vi "Chain4.vi"(7 "Name (\"\" to Use UUID)":string="CSM-Module") -> ()   [LabVIEW 2017, in "CSM-Testcase.lvlib"]
doc: "Creates a template for a CSM module without a user interface.\n\n> [!NOTE] CSM Name Rules\n> - The CSM module name must be unique to avoid entering the \"Critical Error\" state.\n> - If the input is \"\", a UUID will be used as the module name. This module will operate in independent mode and will not be listed in the module list.\n> - If the input ends with '#', the module will run in work mode. Modules with the same name will share the same message queue. External messages will be handled by the idle module.\n\n> [!NOTE] CSM Initialization State\n> - The default value is \"Macro: Initialize\", consistent with the JKISM state machine.\n> - This state is typically not modified and is provided to facilitate external programmatic changes to the initialization state.\n\n\n-- <b>Controls</b> --\n- <b>Name (\"\" to Use UUID)</b>: CSM Module Name\n- <b>Init State(\"Macro: Initialize\")</b>: Initialization State, default is \"Macro: Initialize\""
uses:
  CSM-Testcase.lvlib
  src/user.lib/_NEVSTOP/Communicable State Machine(CSM)/AdvanceAPI/CSM - Revert Arguments-Safe String.vi
  src/user.lib/_NEVSTOP/Communicable State Machine(CSM)/_Shared/Trim Single-line Text.vi
  src/user.lib/_NEVSTOP/Communicable State Machine(CSM)/AdvanceAPI/CSM - Make String Arguments Safe.vi
  src/user.lib/_NEVSTOP/Communicable State Machine(CSM)/AdvanceAPI/CSM - Break Down Multiple States String.vi
  src/user.lib/_NEVSTOP/Communicable State Machine(CSM)/AdvanceAPI/CSM - Keywords.vi
  src/user.lib/_NEVSTOP/Communicable State Machine(CSM)/_Polymophic/Build No-Reply Asynchronous Message with Arguments.vi
  src/user.lib/_NEVSTOP/Communicable State Machine(CSM)/_Polymophic/Build Asynchronous Message with Arguments.vi
  src/user.lib/_NEVSTOP/Communicable State Machine(CSM)/_Polymophic/Build Register Message.vi
  src/user.lib/_NEVSTOP/Communicable State Machine(CSM)/_Polymophic/Build Interrupt Broadcast Message.vi
  src/user.lib/_NEVSTOP/Communicable State Machine(CSM)/Communicable State Machine.lvlib
panel:
  out "Error Occurred":errorcluster
  out "State History":string
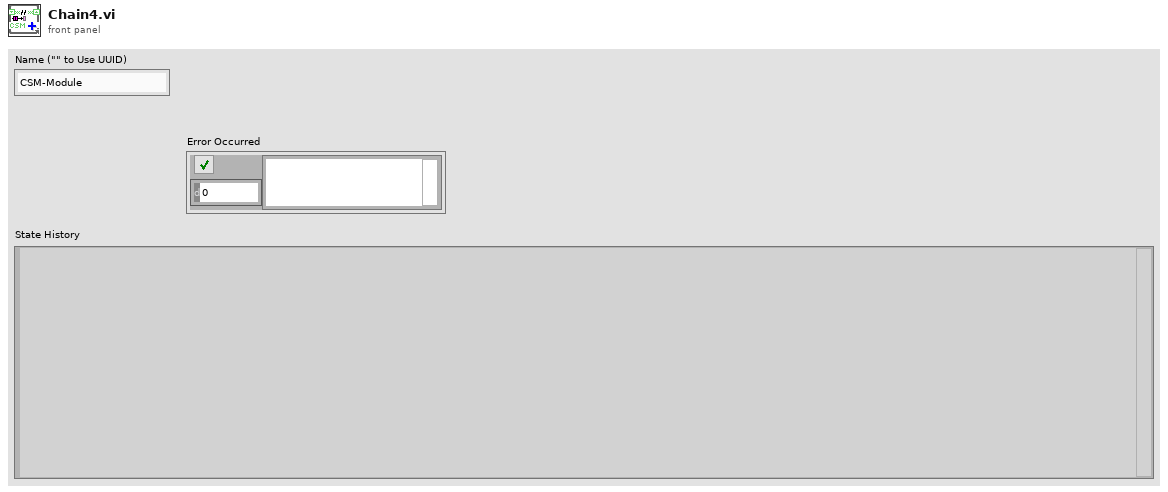
[diagram p1: front panel]
types:
  T1 = cluster{"Arguments":string, "Response":string, "error":errorcluster}
  T2 = enum32{"Invalid", "Standard", "Closed", "Hidden", "Minimized", "Maximized"}
  T3 = enum32{"invalid app kind", "Development System", "Run Time System", "Student Edition", "Embedded LabVIEW", "Evaluation", "Custom"}
  T4 = typedef "Communicable State Machine.lvlib/_CSM_Response Source Message.ctl" = cluster{"‘State":string, "’Arguments":string, "’Error":errorcluster}
  T5 = cluster{"Current VI Reference":refnum<vi>, "Close Panel on Exit?":bool}
  T6 = cluster{"Core":cluster{"Current VI Reference":refnum<vi>, "Close Panel on Exit?":bool}, "Your Boolean data":bool, "Your string data":string, "Counter":u32}
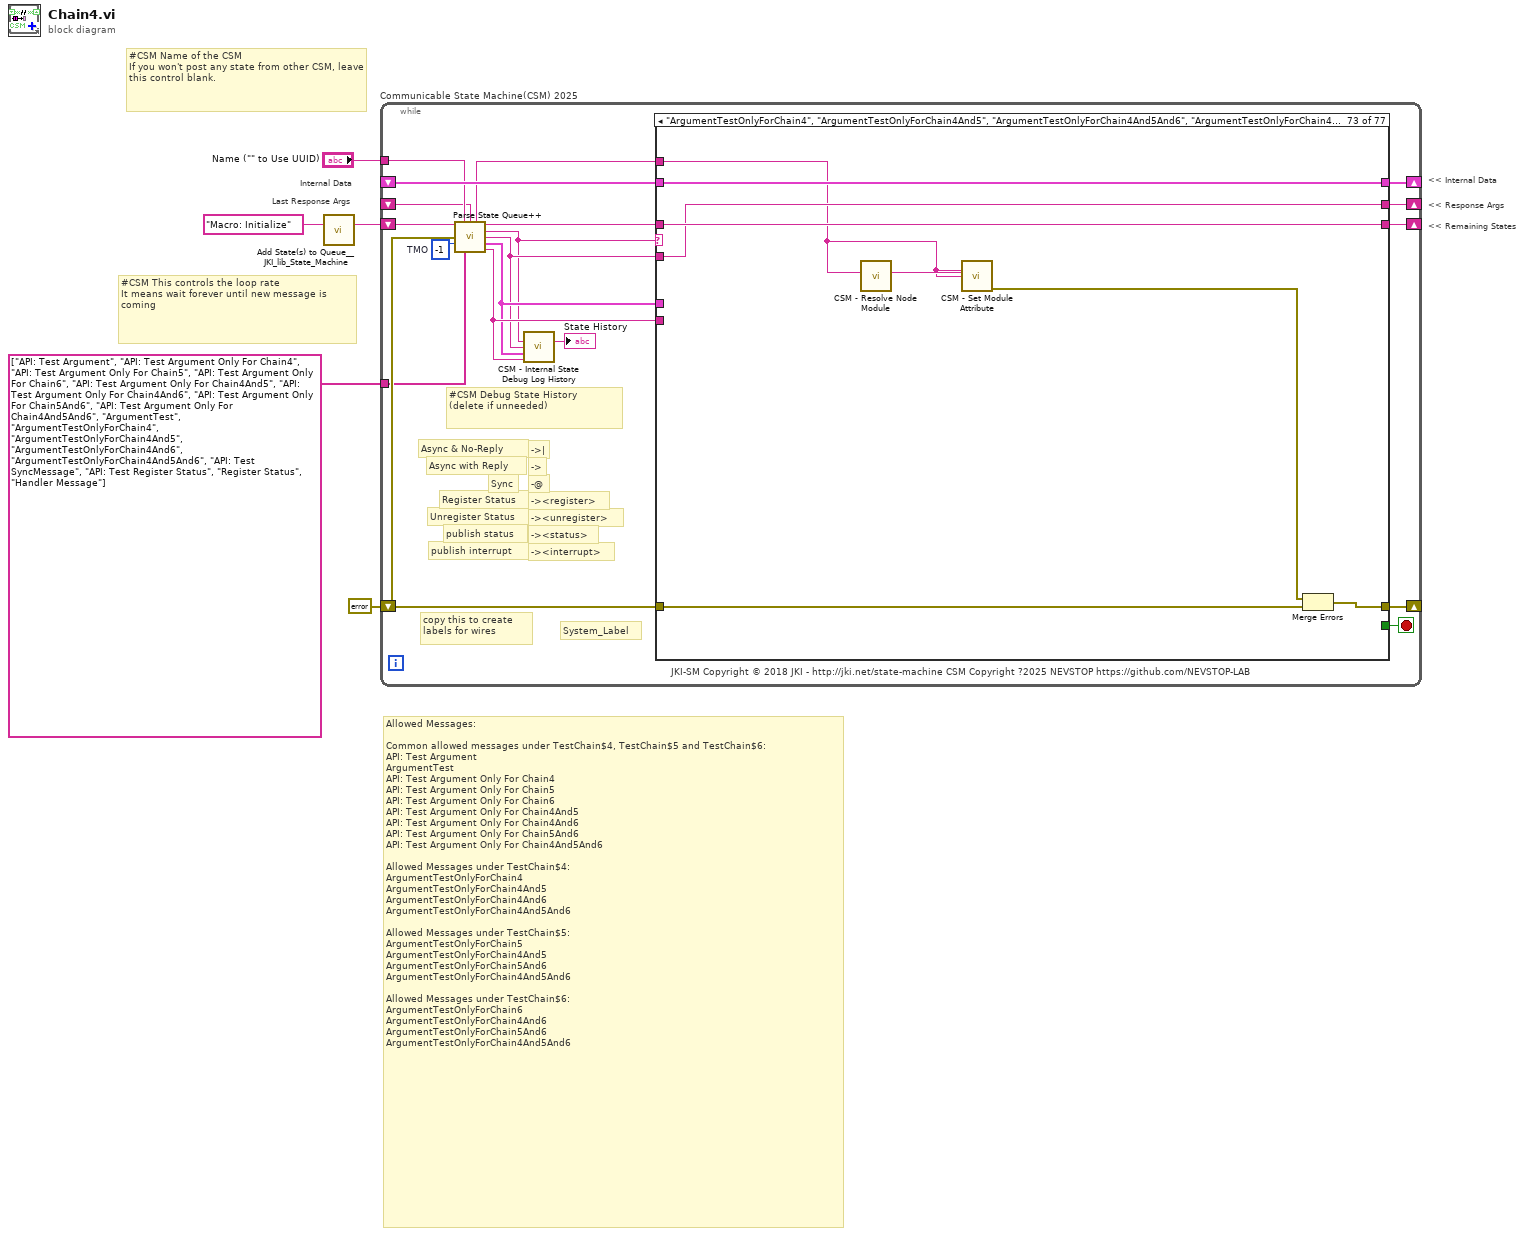
[diagram p0: block diagram]
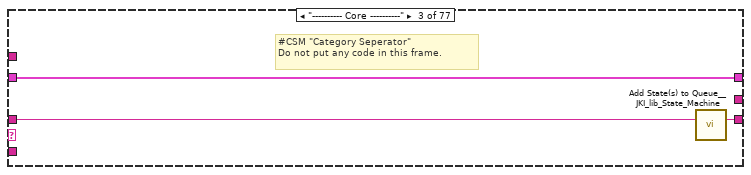
[diagram p4: hidden frame]
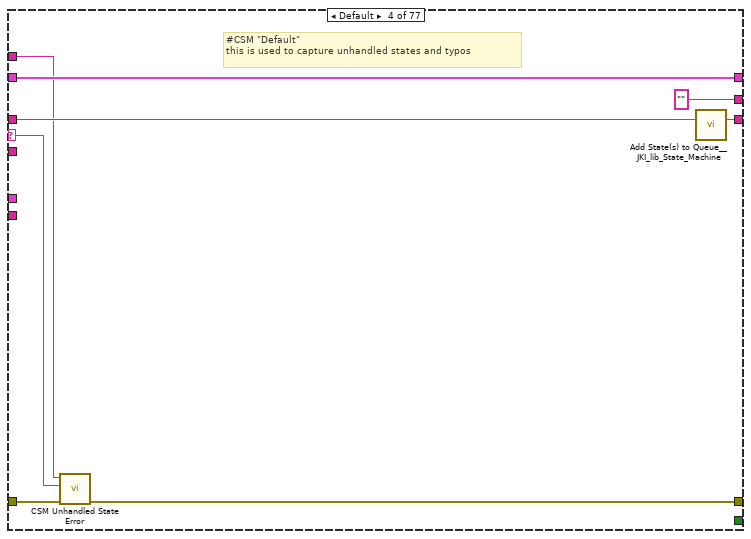
[diagram p5: hidden frame]
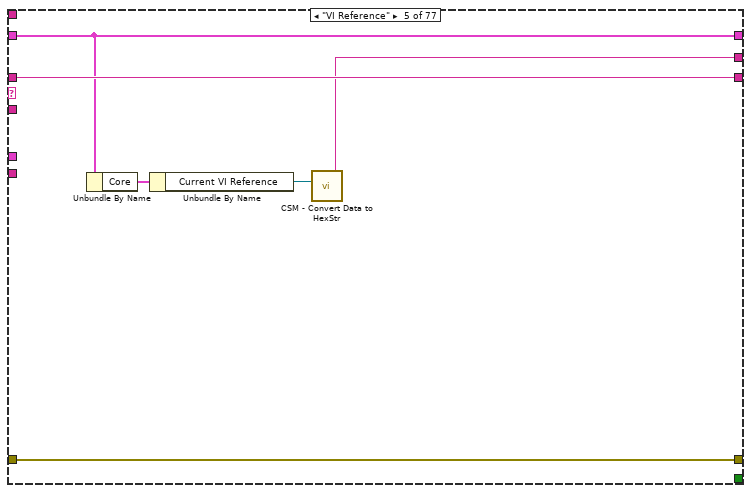
[diagram p6: hidden frame]
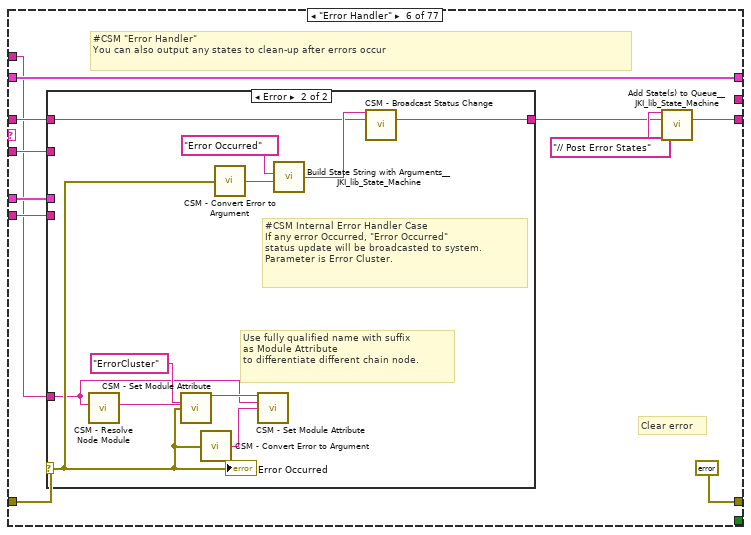
[diagram p7: hidden frame]
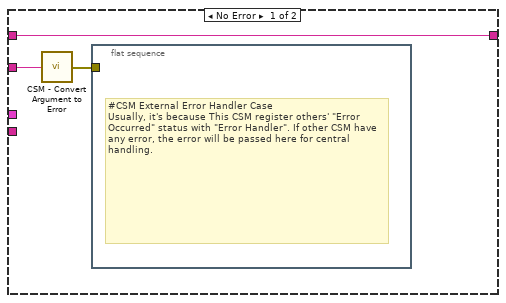
[diagram p8: hidden frame]
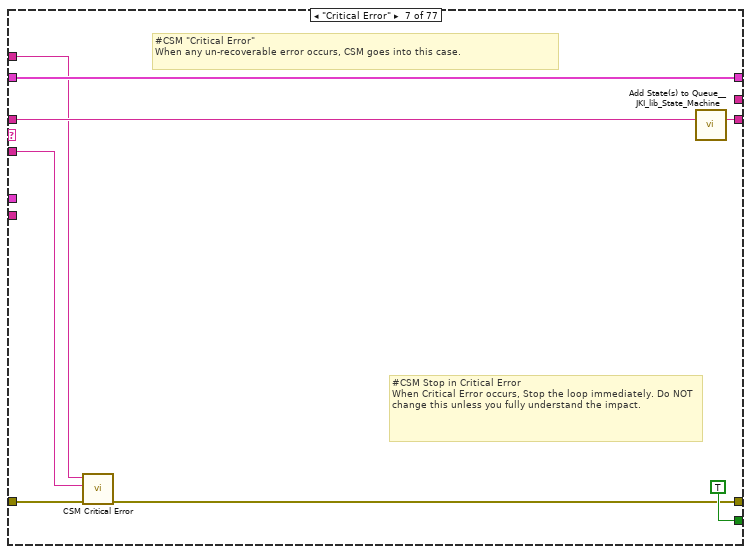
[diagram p9: hidden frame]
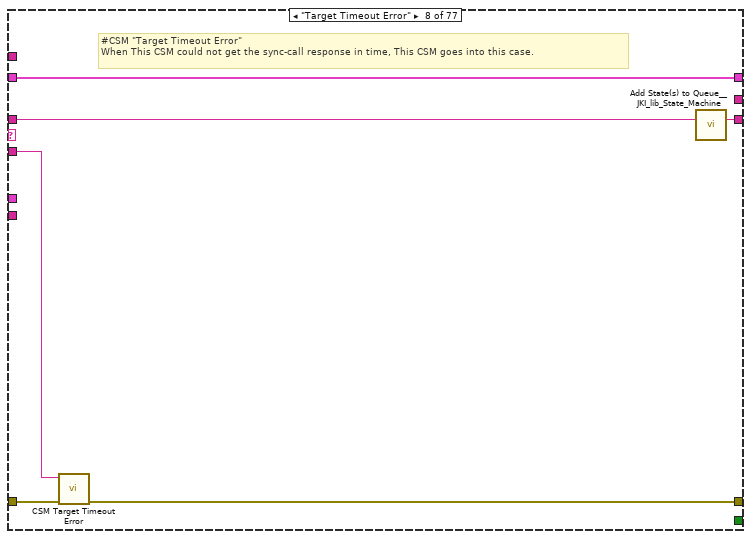
[diagram p10: hidden frame]
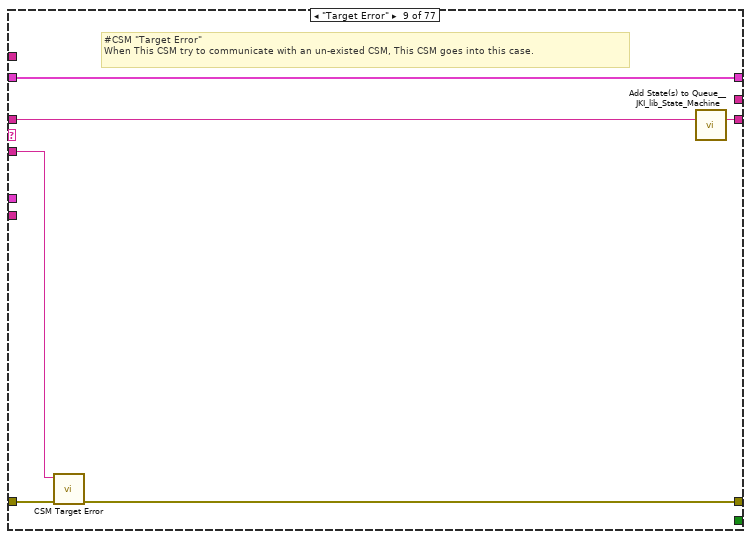
[diagram p11: hidden frame]
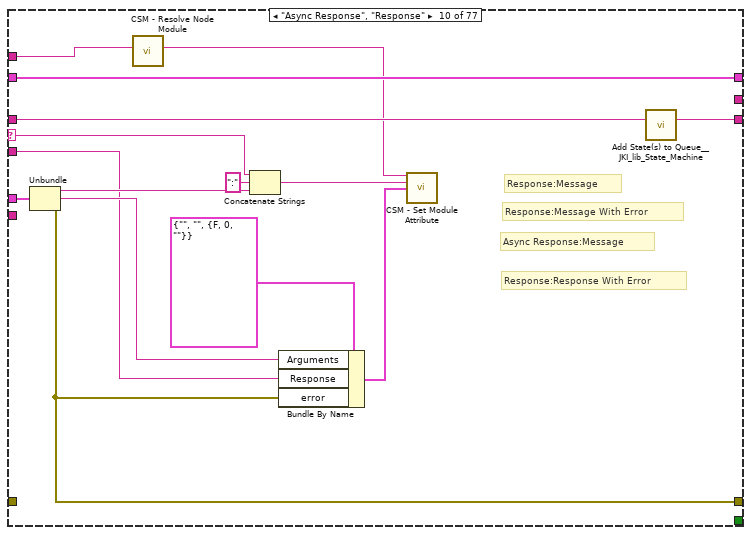
[diagram p12: hidden frame]
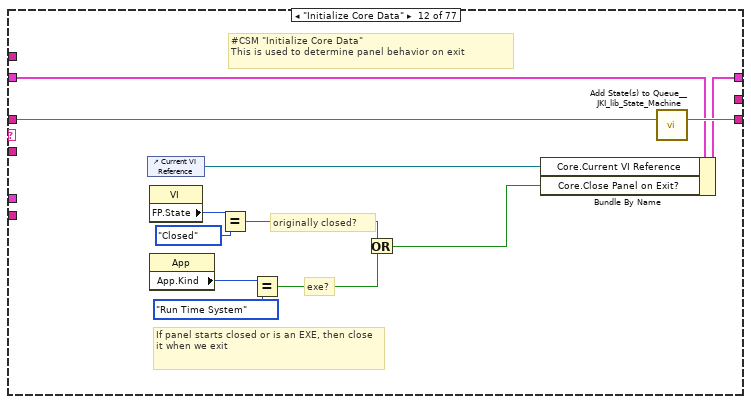
[diagram p14: hidden frame]
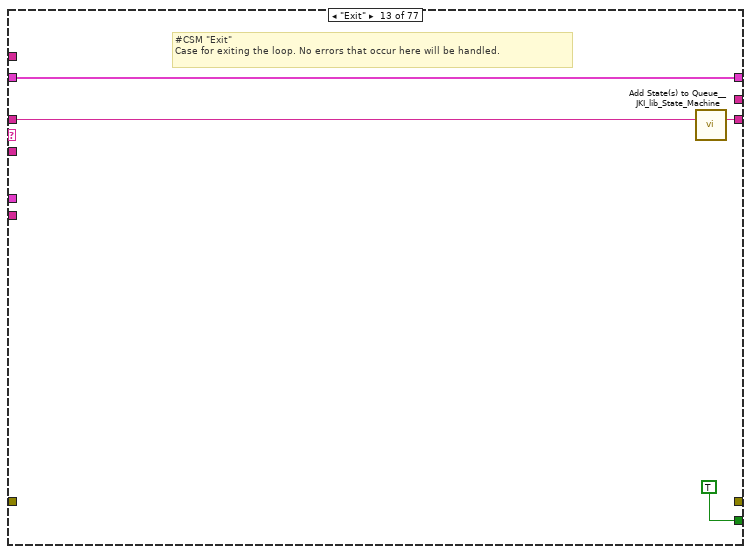
[diagram p15: hidden frame]
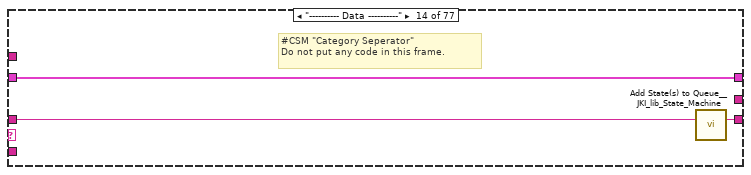
[diagram p16: hidden frame]
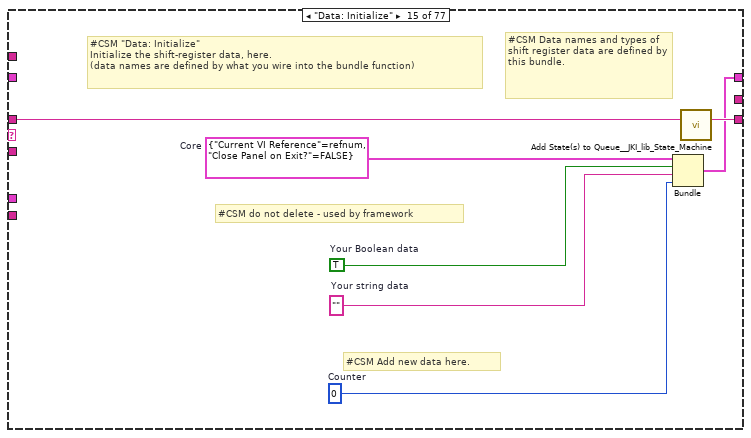
[diagram p17: hidden frame]
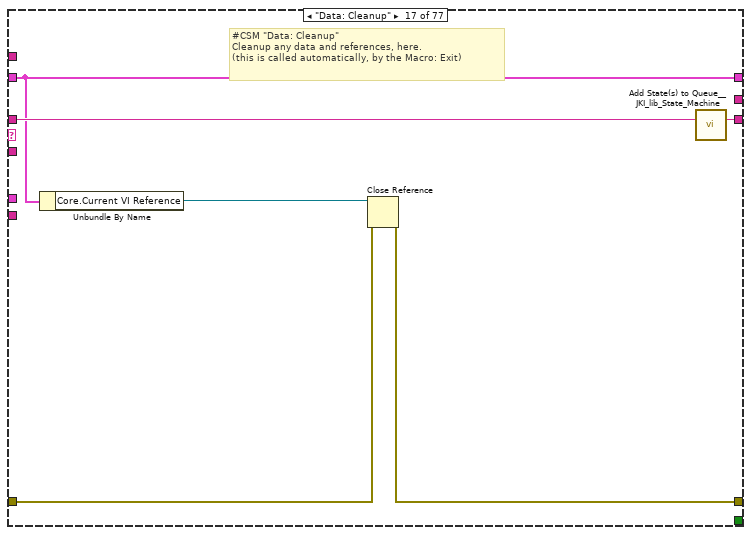
[diagram p19: hidden frame]
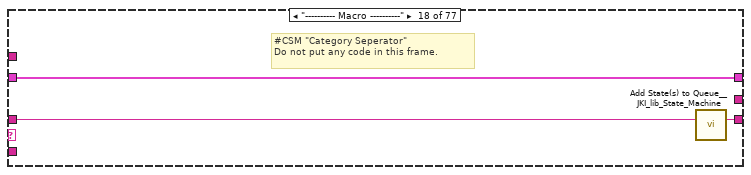
[diagram p20: hidden frame]
diagram:
  # "Allowed Messages:\n\nCommon allowed messages under TestChain$4, TestChain$5 and TestChain$6:\nAPI: Test Argument\nArgumentTest\nAPI: Test Argument Only For Chain4\nAPI: Test Argument Only For Chain5\nAPI: Test Argument Only For Chain6\nAPI: Test Argument Only For Chain4And5\nAPI: Test Argument Only For Chain4And6\nAPI: Test Argument Only For Chain5And6\nAPI: Test Argument Only For Chain4And5And6\n\nAllowed Messages under TestChain$4:\nArgumentTestOnlyForChain4\nArgumentTestOnlyForChain4And5\nArgumentTestOnlyForChain4And6\nArgumentTestOnlyForChain4And5And6\n\nAllowed Messages under TestChain$5:\nArgumentTestOnlyForChain5\nArgumentTestOnlyForChain4And5\nArgumentTestOnlyForChain5And6\nArgumentTestOnlyForChain4And5And6\n\nAllowed Messages under TestChain$6:\nArgumentTestOnlyForChain6\nArgumentTestOnlyForChain4And6\nArgumentTestOnlyForChain5And6\nArgumentTestOnlyForChain4And5And6"
  # "Last Response Args"
  # "Internal Data"
  # "#CSM Name of the CSM\nIf you won't post any state from other CSM, leave this control blank."
  # "#CSM This controls the loop rate\nIt means wait forever until new message is coming"
  # "<< Internal Data"
  # "<< Response Args"
  # "<< Remaining States"
  n1 = call <vilib>:"Add State(s) to Queue__JKI_lib_State_Machine.vi"("State(s) in (\"\")"="Macro: Initialize" ("Init State(\"Macro: Initialize\")")) -> ("States Out"=w5:string)  [unwired: 14 in]
  n2 = while "Communicable State Machine(CSM) 2025" {
    shift-right: [w19] -> _
    shift-left: _ -> [w18]
    shift-right: [w22] -> _
    shift-left: errorcluster {"status"=FALSE, "code"=0, "source"=""} ("error out") -> [w8]
    shift-right: [w21] -> _
    shift-left: w5 -> [w23]
    tunnel: "Name (\"\" to Use UUID)" -> [w15]
    shift-right: [w16] -> _
    shift-left: _ -> [w10]
    tunnel: string[] ["API: Test Argument", "API: Test Argument Only For Chain4", "API: Test Argument Only For Chain5", "API: Test Argument Only For Chain6", "API: Test Argument Only For Chain4And5", "API: Test Argument Only For Chain4And6", "API: Test Argument Only For Chain5And6", "API: Test Argument Only For Chain4And5And6", "ArgumentTest", "ArgumentTestOnlyForChain4", "ArgumentTestOnlyForChain4And5", "ArgumentTestOnlyForChain4And6", "ArgumentTestOnlyForChain4And5And6", "API: Test SyncMessage", "API: Test Register Status", "Register Status", "Handler Message"] ("Allowed Messages (Empty for All)") -> [w6]
    stop <- w20 stop-if-true
    w17 = -1  # TMO
    # "#CSM Debug State History\n(delete if unneeded)"
    # "-><interrupt>"
    # "-><status>"
    # "-><unregister>"
    # "-><register>"
    # "-@"
    # "->"
    # "->|"
    # "publish interrupt"
    # "publish status"
    # "Unregister Status"
    # "Register Status"
    # "Sync"
    # "Async with Reply"
    # "Async & No-Reply"
    # "JKI-SM Copyright © 2018 JKI - http://jki.net/state-machine CSM Copyright ?2025 NEVSTOP https://github.com/NEVSTOP-LAB"
    # "copy this to create labels for wires"
    # "System_Label"
    n3 = call "Parse State Queue++.vi"("State Queue"=w23, "Name (\"\" to Use UUID)"=w15, "Response Arguments"=w10, "Previous Error"=w8, "Dequeue (1 ms)"=w17, "Allowed Messages (Empty for All)"=w6) -> ("Name Used"=w9:string, "Remaining States"=w24:string, "Current State"=w11:string, "Arguments"=w12:string, "Additional Information"=w13:T4, "Source CSM"=w14:string)  [unwired: 4 in]
    n4 = call "CSM - Internal State Debug Log History.vi"("State"=w11, "Arguments (\"\")"=w12, ">> Response Source Message >>"=w13, "Source (\"\")"=w14) -> ("Debug Log"=→"State History":string)  [unwired: 11 in]
    n5 = case shown="\"ArgumentTestOnlyForChain4\", \"ArgumentTestOnlyForChain4And5\", \"ArgumentTestOnlyForChain4And5And6\", \"ArgumentTestOnlyForChain4And6\", \"ArgumentTestOnlyForChain5\", \"ArgumentTestOnlyForChain5And6\", \"ArgumentTestOnlyForChain6\"" w11 {
      selector: w11 -> [_ _ _ w35 _ _ _ _ _ w101 _ _ _ _ _ _ _ _ _ _ _ _ _ _ _ _ _ _ _ _ _ _ _ w380 _ _ _ _ _ _ _ _ _ _ _ _ _ _ _ _ _ _ _ _ _ _ w567 _ _ _ _ _ _ _ _ _ _ w633 _ _ _ w657 _ w676 w683 w698 _]
      tunnel: w24 -> [w25 w28 w31 w39 w44 w50 w78 w84 w90 w105 w107 w119 w123 w126 w133 w135 w141 w144 w148 w154 w168 w188 w217 w221 w225 w237 w262 w290 w305 w317 w329 w343 w366 w398 w414 w427 w434 w441 w448 w455 w462 w469 w476 w483 w490 w497 w504 w515 w523 w532 w541 w550 w554 w559 w562 w566 w572 w579 w582 w594 w600 w606 w610 w615 w619 w623 w627 w636 w640 w648 w654 w661 w670 w678 w687 w702 w712]
      tunnel: w12 -> [_ _ _ _ _ w49 w74 w81 w87 w95 _ _ _ _ _ _ _ _ _ _ w155 w175 w200 _ w228 w240 w265 w293 w308 w320 w332 w346 w362 w396 w417 w424 w431 w438 w445 w452 w459 w466 w473 w480 w487 w494 w501 w508 _ w525 w533 w542 w552 _ _ w563 _ w575 w584 _ w596 w602 w608 w613 w618 w622 w626 w632 w639 w646 w652 w658 w667 w677 w682 w693 _]
      tunnel: w18 -> [w26 w27 w29 w37 w43 w55 w76 w82 w88 w103 w106 w113 w121 w124 _ w134 w136 w142 w146 w152 w170 w190 w219 w220 w229 w241 w266 w294 w309 w321 w333 w347 w369 w401 w418 w429 w436 w443 w450 w457 w464 w471 w478 w485 w492 w499 w506 w513 w521 w530 w539 w548 w553 w557 w560 w564 w573 w580 w586 w595 w601 w607 w612 w617 w620 w624 w628 w637 w641 w647 w653 w662 w665 w679 w688 w695 w710]
      tunnel: [_ _ _ w32 w45 errorcluster {"status"=FALSE, "code"=0, "source"=""} ("error out") w71 w79 w85 w94 _ _ _ _ _ _ w137 _ _ _ _ _ _ _ w222 w234 w259 w287 w302 w314 w326 w339 w363 w382 w411 w428 w435 w442 w449 w456 w463 w470 w477 w484 w491 w498 w505 _ _ _ w537 w546 _ _ _ _ _ _ _ _ _ _ w611 w616 w621 w625 w629 w631 w642 w643 w649 w656 w668 w673 w684 w699 _] -> w22
      tunnel: w8 -> [_ _ _ w33 w45 w53 w72 w80 w86 _ _ _ _ _ _ _ w138 _ _ _ _ _ _ _ _ _ _ _ _ _ _ _ _ _ _ w428 w435 w442 w449 w456 w463 w470 w477 w484 w491 w498 w505 _ _ _ _ _ _ _ _ _ _ _ _ _ _ _ w611 w616 w621 w625 w629 w638 w642 w644 w650 w663 w671 w680 w689 w703 _]
      tunnel: [w25 w28 w30 w38 w44 w51 w77 w83 w89 w104 w107 w118 w122 w125 w132 w135 w140 w143 w147 w153 w169 w189 w218 w221 w226 w238 w263 w291 w306 w318 w330 w344 w367 w399 w415 w426 w433 w440 w447 w454 w461 w468 w475 w482 w489 w496 w503 w514 w522 w531 w540 w549 w554 w558 w561 w565 w574 w576 w581 w592 w597 w603 w609 w614 w619 w623 w627 w636 w640 w648 w654 w661 w670 w678 w687 w702 w711] -> w21
      tunnel: [_ _ _ _ _ _ TRUE _ _ _ _ _ TRUE _ _ _ _ _ _ _ _ _ _ _ _ _ _ _ _ _ _ _ _ _ _ _ _ _ _ _ _ _ _ _ _ _ _ _ _ _ _ _ _ _ _ _ _ _ _ _ _ _ _ _ _ _ _ _ _ _ _ _ _ _ _ _ _] -> w20
      tunnel: [w26 w27 w29 w37 w43 w55 w76 w82 w88 w103 w106 w117 w121 w124 w131 w134 w136 w142 w146 w152 w170 w190 w219 w220 w229 w241 w266 w294 w309 w321 w333 w347 w369 w401 w418 w429 w436 w443 w450 w457 w464 w471 w478 w485 w492 w499 w506 w513 w521 w530 w539 w548 w553 w557 w560 w564 w573 w580 w586 w595 w601 w607 w612 w617 w620 w624 w628 w637 w641 w647 w653 w662 w665 w679 w688 w694 w708] -> w19
      tunnel: w14 -> [_ _ _ _ _ w48 _ _ _ _ _ _ _ _ _ _ _ _ _ _ _ _ _ _ _ _ _ _ _ _ _ _ _ _ _ _ _ _ _ _ _ _ _ _ _ _ _ _ _ _ _ _ _ _ _ _ _ _ _ _ _ _ _ _ _ _ _ _ _ _ _ _ _ _ _ _ _]
      tunnel: w13 -> [_ _ _ _ _ w47 _ _ _ w102 _ _ _ _ _ _ _ _ _ _ _ _ _ _ _ _ _ _ _ _ _ _ _ _ _ _ _ _ _ _ _ _ _ _ _ _ _ _ _ _ _ _ _ _ _ _ _ _ _ _ _ _ _ _ _ _ _ _ _ _ _ _ _ _ _ _ _]
      tunnel: [_ _ _ "" w40 _ _ _ _ _ _ _ _ _ _ _ _ _ _ _ _ _ _ _ _ _ _ _ _ _ _ _ _ w383 _ _ _ _ _ _ _ _ _ _ _ _ _ _ _ _ _ _ w551 _ _ w563 w568 _ _ _ _ _ w608 w613 w618 w622 w626 w632 w639 w646 w652 _ w667 w677 w682 _ _] -> w16
      tunnel: w9 -> [_ _ _ w34 _ w46 w73 _ _ w92 _ _ _ _ _ _ _ _ _ _ _ _ _ _ _ _ w250 w278 _ _ _ w340 _ w386 _ _ _ _ _ _ _ _ _ _ _ _ _ w511 w519 w528 w538 w547 _ _ _ _ w569 _ _ w589 _ _ _ _ _ _ _ w635 _ _ _ w660 w664 w675 w686 w701 _]
      frame "", "Idle" {
        # "#CSM \"Idle/Event Handler\"\nexecutes when the state queue is empty"
      }
      frame "CSM Documentation" {
        # "#CSM State Syntax\n\n// Comment line, all text to the right of “//” will be ignored\n// Local Message Example\nDoSth: DoA >> Arguments\n\n// Sync Call Example\nAPI: xxxx >> Arguments -@ TargetModule\n\n// Async Call Example\nAPI: xxxx >> Arguments -> TargetModule\n\n// Async Call without Reply Example\nAPI: xxxx >> Arguments ->| TargetModule\n\n// Broadcast normal status:\nStatus >> StatusArguments  -><status>\n\n// Broadcast Interrupt status:\nInterrupt >> StatusArguments  -><interrupt>\n\n// Register Source Module's status to Handler Module\nStatus@Source Module >> Handler Module@Handler Module -><register>\n\n// Unegister Source Module's status\nStatus@Source Module >> Handler Module -><unregister>"
        # "#CSM README FIRST\n\nCommunicable State Machine(CSM) is a LabVIEW application framework that builds upon JKI State Machine(JKISM). It follows the pattern of JKISM and extends the keywords to describe message communication between modules, including concepts such as Sync-Message, Async-Message, Subscription/Unsubscription of status - essential elements for creating reusable code modules. For more information, please visit the CSM wiki: https://nevstop-lab.github.io/CSM-Wiki/\n\nFor instructions on JKI State Machine, visit: \n    http://jki.net/state-machine/\nFor information about CSM, visit: \n    https://github.com/NEVSTOP-LAB"
        # "#CSM \"Documentation\"\nCase for holding CSM Documenation"
      }
      frame "---------- Core ----------" {
        # "#CSM \"Category Seperator\"\nDo not put any code in this frame."
        n6 = call <vilib>:"Add State(s) to Queue__JKI_lib_State_Machine.vi"("State(s) in (\"\")"=w31) -> ("States Out"=w30:string)  [unwired: 14 in]
      }
      frame Default {
        # "#CSM \"Default\"\nthis is used to capture unhandled states and typos"
        n7 = call "CSM Unhandled State Error.vi"("error in (no error)"=w33, "Undefined State"=w35, "CSM Name"=w34) -> ("error out"=w32:errorcluster)  [unwired: 8 in]
        n8 = call <vilib>:"Add State(s) to Queue__JKI_lib_State_Machine.vi"("State(s) in (\"\")"=w39) -> ("States Out"=w38:string)  [unwired: 14 in]
      }
      frame "VI Reference" {
        n9 = Unbundle By Name(w43) -> ("Core"=w42:T5)
        n10 = Unbundle By Name(w42) -> ("Current VI Reference"=w41:refnum<vi>)
        n11 = call "CSM - Convert Data to HexStr.vi"("Variant"=w41) -> ("HEX String (0-9,A-F)"=w40:string)  [unwired: 8 in]
      }
      frame "Error Handler" {
        # "#CSM \"Error Handler\"\nYou can also output any states to clean-up after errors occur"
        # "Clear error"
        n12 = case shown="Error" w53 {
          selector: w53 -> [_ w62]
          tunnel: [w59 w67] -> w52
          tunnel: w50 -> [w59 w66]
          tunnel: w49 -> [w58 _]
          tunnel: w48 -> [_ _]
          tunnel: w47 -> [_ _]
          tunnel: w46 -> [_ w60]
          frame No Error {
            n13 = call "CSM - Convert Argument to Error.vi"("Argument"=w58) -> ("Error"=w57:errorcluster)  [unwired: 4 in]
            n14 = flat-sequence {
              tunnel: w57 -> [_]
              frame #0 {
                # "#CSM External Error Handler Case\nUsually, it's because This CSM register others' \"Error Occurred\" status with \"Error Handler\". If other CSM have any error, the error will be passed here for central handling."
              }
            }
          }
          frame Error {
            # "Use fully qualified name with suffix \nas Module Attribute  \nto differentiate different chain node."
            # "#CSM Internal Error Handler Case \nIf any error Occurred, \"Error Occurred\" \nstatus update will be broadcasted to system.\nParameter is Error Cluster."
            n15 = call "CSM - Resolve Node Module.vi"("Node Name"=w60) -> ("CSM Module Name"=w65:string)  [unwired: 10 in]
            n16 = call "CSM - Set Module Attribute.vi"("CSM Name"=w65, "Attribute"="ErrorCluster", "Value"=w62) -> ("CSM Name (Dup)"=w63:string)  [unwired: 9 in, 3 out]
            n17 = call "CSM - Convert Error to Argument.vi"("Error"=w62) -> ("Argument"=w61:string)  [unwired: 4 in]
            n18 = call "CSM - Convert Error to Argument.vi"("Error"=w62) -> ("Argument"=w69:string)  [unwired: 4 in]
            n19 = call "CSM - Set Module Attribute.vi"("CSM Name"=w63, "Attribute"=w60, "Value"=w61) -> ()  [unwired: 9 in, 4 out]
            n20 = call <vilib>:"Build State String with Arguments__JKI_lib_State_Machine.vi"("Arguments (\"\")"=w69, "State"="Error Occurred" ("Status with Arguments")) -> ("State with Arguments"=w68:string)  [unwired: 4 in]
            n21 = call "CSM - Broadcast Status Change.vi"("Status With Arguments"=w68, "State Queue"=w66) -> ("Remaining States"=w67:string)  [unwired: 13 in]
            "Error Occurred" <- w62
          }
        }
        n22 = call <vilib>:"Add State(s) to Queue__JKI_lib_State_Machine.vi"("State(s) in Front (\"\")"="// Post Error States", "State(s) in (\"\")"=w52) -> ("States Out"=w51:string)  [unwired: 13 in]
      }
      frame "Critical Error" {
        # "#CSM \"Critical Error\"\nWhen any un-recoverable error occurs, CSM goes into this case."
        # "#CSM Stop in Critical Error\nWhen Critical Error occurs, Stop the loop immediately. Do NOT change this unless you fully understand the impact."
        n23 = call "CSM Critical Error.vi"("error in (no error)"=w72, "Arugments (As Reason)"=w74, "CSM Name"=w73) -> ("error out"=w71:errorcluster)  [unwired: 8 in]
        n24 = call <vilib>:"Add State(s) to Queue__JKI_lib_State_Machine.vi"("State(s) in (\"\")"=w78) -> ("States Out"=w77:string)  [unwired: 14 in]
      }
      frame "Target Timeout Error" {
        # "#CSM \"Target Timeout Error\"\nWhen This CSM could not get the sync-call response in time, This CSM goes into this case."
        n25 = call "CSM Target Timeout Error.vi"("error in (no error)"=w80, "Arguments (As CSM Name)"=w81) -> ("error out"=w79:errorcluster)  [unwired: 9 in]
        n26 = call <vilib>:"Add State(s) to Queue__JKI_lib_State_Machine.vi"("State(s) in (\"\")"=w84) -> ("States Out"=w83:string)  [unwired: 14 in]
      }
      frame "Target Error" {
        # "#CSM \"Target Error\"\nWhen This CSM try to communicate with an un-existed CSM, This CSM goes into this case."
        n27 = call "CSM Target Error.vi"("error in (no error)"=w86, "Arguments (As CSM Name)"=w87) -> ("error out"=w85:errorcluster)  [unwired: 9 in]
        n28 = call <vilib>:"Add State(s) to Queue__JKI_lib_State_Machine.vi"("State(s) in (\"\")"=w90) -> ("States Out"=w89:string)  [unwired: 14 in]
      }
      frame "Async Response", "Response" {
        # "Response:Response With Error"
        # "Response:Message With Error"
        # "Async Response:Message"
        # "Response:Message"
        n29 = Unbundle(w102) -> ("‘State"=w100:string, "’Arguments"=w96:string, "’Error"=w94:errorcluster)
        n30 = call "CSM - Resolve Node Module.vi"("Node Name"=w92) -> ("CSM Module Name"=w91:string)  [unwired: 10 in]
        n31 = Concatenate Strings(w101, ":" ("string"), w100) -> (w98:string)
        n32 = Bundle By Name(cluster=T1 {"Arguments"="", "Response"="", "error"={"status"=FALSE, "code"=0, "source"=""}}, "Arguments"=w96, "Response"=w95, "error"=w94) -> (w93:T1)
        n33 = call "CSM - Set Module Attribute.vi"("CSM Name"=w91, "Attribute"=w98, "Value"=w93) -> ()  [unwired: 9 in, 4 out]
        n34 = call <vilib>:"Add State(s) to Queue__JKI_lib_State_Machine.vi"("State(s) in (\"\")"=w105) -> ("States Out"=w104:string)  [unwired: 14 in]
      }
      frame "Async Message Posted" {
        # "#CSM \"Async Message Posted\"\nAfter Async Message is posted (-> or ->| ), CSM goes to this state for post-action.\nYou can use Argument - State to tell which Async Message is called."
      }
      frame "Initialize Core Data" {
        # "#CSM \"Initialize Core Data\"\nThis is used to determine panel behavior on exit"
        # "originally closed?"
        # "exe?"
        # "If panel starts closed or is an EXE, then close it when we exit"
        n35 = control-ref of="Current VI Reference"() -> (w111:refnum<vi>)
        n36 = property class="VI"() -> ("FP.State"=w110:T2)  [unwired: 2 in, 2 out]
        n37 = property class="App"() -> ("App.Kind"=w116:T3)  [unwired: 2 in, 2 out]
        n38 = Equal?(x=w110, y=T2."Closed" ("Front Panel Window:State")) -> (x = y?=w108:bool)
        n39 = Equal?(x=w116, y=T3."Run Time System" ("Application:Kind")) -> (x = y?=w114:bool)
        n40 = Or(x=w108, y=w114) -> (x .or. y?=w112:bool)
        n41 = Bundle By Name(cluster=w113, "Core.Current VI Reference"=w111, "Core.Close Panel on Exit?"=w112) -> (w117:T6)
        n42 = call <vilib>:"Add State(s) to Queue__JKI_lib_State_Machine.vi"("State(s) in (\"\")"=w119) -> ("States Out"=w118:string)  [unwired: 14 in]
      }
      frame "Exit" {
        # "#CSM \"Exit\"\nCase for exiting the loop. No errors that occur here will be handled."
        n43 = call <vilib>:"Add State(s) to Queue__JKI_lib_State_Machine.vi"("State(s) in (\"\")"=w123) -> ("States Out"=w122:string)  [unwired: 14 in]
      }
      frame "---------- Data ----------" {
        # "#CSM \"Category Seperator\"\nDo not put any code in this frame."
        n44 = call <vilib>:"Add State(s) to Queue__JKI_lib_State_Machine.vi"("State(s) in (\"\")"=w126) -> ("States Out"=w125:string)  [unwired: 14 in]
      }
      frame "Data: Initialize" {
        w127 = u32 0  # Counter
        w128 = T5 {"Current VI Reference"=refnum, "Close Panel on Exit?"=FALSE}  # Core
        w130 = TRUE  # Your Boolean data
        w129 = ""  # Your string data
        # "#CSM \"Data: Initialize\"\nInitialize the shift-register data, here.\n(data names are defined by what you wire into the bundle function)"
        # "#CSM do not delete - used by framework"
        # "#CSM Add new data here."
        # "#CSM Data names and types of shift register data are defined by this bundle."
        n45 = Bundle("Core"=w128, "Your Boolean data"=w130, "Your string data"=w129, "Counter"=w127) -> (w131:T6)  [unwired: 1 in]
        n46 = call <vilib>:"Add State(s) to Queue__JKI_lib_State_Machine.vi"("State(s) in (\"\")"=w133) -> ("States Out"=w132:string)  [unwired: 14 in]
      }
      frame "Data: Update Indicators" {
      }
      frame "Data: Cleanup" {
        # "#CSM \"Data: Cleanup\"\nCleanup any data and references, here.\n(this is called automatically, by the Macro: Exit)"
        n47 = Unbundle By Name(w136) -> ("Core.Current VI Reference"=w139:refnum<vi>)
        n48 = Close Reference(reference=w139, error in (no error)=w138) -> (error out=w137:errorcluster)
        n49 = call <vilib>:"Add State(s) to Queue__JKI_lib_State_Machine.vi"("State(s) in (\"\")"=w141) -> ("States Out"=w140:string)  [unwired: 14 in]
      }
      frame "---------- Macro ----------" {
        # "#CSM \"Category Seperator\"\nDo not put any code in this frame."
        n50 = call <vilib>:"Add State(s) to Queue__JKI_lib_State_Machine.vi"("State(s) in (\"\")"=w144) -> ("States Out"=w143:string)  [unwired: 14 in]
      }
      frame "Macro: Initialize" {
        # "#CSM \"Macro: Initialize\"\nInitialization Macro (This is called once, when the VI starts)"
        n51 = call <vilib>:"Add State(s) to Queue__JKI_lib_State_Machine.vi"("State(s) in Front (\"\")"="Data: Initialize\nInitialize Core Data\nData: Update Indicators", "State(s) in (\"\")"=w148) -> ("States Out"=w147:string)  [unwired: 13 in]
      }
      frame "Macro: Exit" {
        # "#CSM \"Macro: Exit\"\nExit Macro (This is called once, when the VI exits)"
        n52 = call <vilib>:"Add State(s) to Queue__JKI_lib_State_Machine.vi"("State(s) in Front (\"\")"="//Exit Sub-Modules ", "State(s) at Back (\"\")"="Data: Cleanup\nExit") -> ("States Out"=w150:string)  [unwired: 13 in]
        n53 = call <vilib>:"Add State(s) to Queue__JKI_lib_State_Machine.vi"("State(s) in Front (\"\")"=w150, "State(s) in (\"\")"=w154) -> ("States Out"=w153:string)  [unwired: 13 in]
      }
      frame "Macro: Test MacroWithSubMessages" {
        w156 = "SubMessage2" ("State With Arguments")
        w158 = "SubMessage1" ("State With Arguments")
        n54 = call "uuid.vi"() -> ("UUID"=w157:string)  [unwired: 11 in]
        n55 = call "uuid.vi"() -> ("UUID"=w159:string)  [unwired: 11 in]
        n56 = Concatenate Strings(w158, w159) -> (w160:string)
        n57 = Concatenate Strings(w156, w157) -> (w161:string)
        n58 = call <vilib>:"Build State String with Arguments__JKI_lib_State_Machine.vi"("Arguments (\"\")"=w155, "State"="SubMessage3" ("State With Arguments")) -> ("State with Arguments"=w163:string)  [unwired: 4 in]
        n59 = call <vilib>:"Build State String with Arguments__JKI_lib_State_Machine.vi"("Arguments (\"\")"=w160, "State"=w158) -> ("State with Arguments"=w165:string)  [unwired: 4 in]
        n60 = call <vilib>:"Build State String with Arguments__JKI_lib_State_Machine.vi"("Arguments (\"\")"=w161, "State"=w156) -> ("State with Arguments"=w164:string)  [unwired: 4 in]
        n61 = Build Array(w165, w164, w163) -> (w162:string[])
        n62 = call "CSM - Compact Multiple States.vi"("Multiple States"=w162) -> ("States"=w167:string)  [unwired: 9 in]
        n63 = call <vilib>:"Add State(s) to Queue__JKI_lib_State_Machine.vi"("State(s) in Front (\"\")"=w167, "State(s) in (\"\")"=w168) -> ("States Out"=w169:string)  [unwired: 13 in]
      }
      frame "Macro: Test MacroWithSubAndPostMessages" {
        w174 = "PostMessage1" ("State With Arguments")
        w176 = "SubMessage2" ("State With Arguments")
        w178 = "SubMessage1" ("State With Arguments")
        n64 = call "uuid.vi"() -> ("UUID"=w177:string)  [unwired: 11 in]
        n65 = call "uuid.vi"() -> ("UUID"=w173:string)  [unwired: 11 in]
        n66 = call "uuid.vi"() -> ("UUID"=w179:string)  [unwired: 11 in]
        n67 = Concatenate Strings(w174, w173) -> (w172:string)
        n68 = Concatenate Strings(w178, w179) -> (w180:string)
        n69 = Concatenate Strings(w176, w177) -> (w181:string)
        n70 = call <vilib>:"Build State String with Arguments__JKI_lib_State_Machine.vi"("Arguments (\"\")"=w175, "State"="SubMessage3" ("State With Arguments")) -> ("State with Arguments"=w183:string)  [unwired: 4 in]
        n71 = call <vilib>:"Build State String with Arguments__JKI_lib_State_Machine.vi"("Arguments (\"\")"=w172, "State"=w174) -> ("State with Arguments"=w171:string)  [unwired: 4 in]
        n72 = call <vilib>:"Build State String with Arguments__JKI_lib_State_Machine.vi"("Arguments (\"\")"=w180, "State"=w178) -> ("State with Arguments"=w185:string)  [unwired: 4 in]
        n73 = call <vilib>:"Build State String with Arguments__JKI_lib_State_Machine.vi"("Arguments (\"\")"=w181, "State"=w176) -> ("State with Arguments"=w184:string)  [unwired: 4 in]
        n74 = Build Array(w185, w184, w183) -> (w182:string[])
        n75 = call "CSM - Compact Multiple States.vi"("Multiple States"=w182) -> ("States"=w187:string)  [unwired: 9 in]
        n76 = call <vilib>:"Add State(s) to Queue__JKI_lib_State_Machine.vi"("State(s) in Front (\"\")"=w187, "State(s) in (\"\")"=w188, "State(s) at Back (\"\")"=w171) -> ("States Out"=w189:string)  [unwired: 12 in]
      }
      frame "Macro: TestMacroWithNonLocalSubMessages" {
        w204 = "PostMessage1" ("State With Arguments")
        w205 = "SubMessage2" ("State With Arguments")
        w207 = "SubMessage1" ("State With Arguments")
        n77 = Match Pattern(string=w200, regular expression="+") -> (before substring=w192:string, after substring=w191:string)  [unwired: 1 in, 2 out]
        n78 = call "uuid.vi"() -> ("UUID"=w203:string)  [unwired: 11 in]
        n79 = call "uuid.vi"() -> ("UUID"=w206:string)  [unwired: 11 in]
        n80 = call "uuid.vi"() -> ("UUID"=w208:string)  [unwired: 11 in]
        n81 = Concatenate Strings(w204, w203) -> (w202:string)
        n82 = Concatenate Strings(w207, w208) -> (w209:string)
        n83 = Concatenate Strings(w205, w206) -> (w210:string)
        n84 = call <vilib>:"Build State String with Arguments__JKI_lib_State_Machine.vi"("Arguments (\"\")"=w202, "State"=w204) -> ("State with Arguments"=w201:string)  [unwired: 4 in]
        n85 = call-poly "Build Message with Arguments++.vi"("State With Arguments"="SubMessage1", "Target Module (\"\")"=w191) -> ("CSM Message String"=w196:string)  [unwired: 13 in]
        n86 = call-poly "Build Message with Arguments++.vi"("State With Arguments"="SubMessage2", "Target Module (\"\")"=w191) -> ("CSM Message String"=w195:string)  [unwired: 13 in]
        n87 = call <vilib>:"Build State String with Arguments__JKI_lib_State_Machine.vi"("Arguments (\"\")"=w192, "State"="SubMessage3" ("State With Arguments")) -> ("State with Arguments"=w212:string)  [unwired: 4 in]
        n88 = call-poly "Build Message with Arguments++.vi"("State With Arguments"="Message", "Target Module (\"\")"=w191) -> ("CSM Message String"=w197:string)  [unwired: 13 in]
        n89 = call <vilib>:"Build State String with Arguments__JKI_lib_State_Machine.vi"("Arguments (\"\")"=w209, "State"=w207) -> ("State with Arguments"=w214:string)  [unwired: 4 in]
        n90 = call <vilib>:"Build State String with Arguments__JKI_lib_State_Machine.vi"("Arguments (\"\")"=w210, "State"=w205) -> ("State with Arguments"=w213:string)  [unwired: 4 in]
        n91 = Build Array(w214, w213, w212, w197, w196, w195) -> (w211:string[])
        n92 = call "CSM - Compact Multiple States.vi"("Multiple States"=w211) -> ("States"=w216:string)  [unwired: 9 in]
        n93 = call <vilib>:"Add State(s) to Queue__JKI_lib_State_Machine.vi"("State(s) in Front (\"\")"=w216, "State(s) in (\"\")"=w217, "State(s) at Back (\"\")"=w201) -> ("States Out"=w218:string)  [unwired: 12 in]
      }
      frame "---------- API ----------" {
        # "#CSM \"Category Seperator\"\nDo not put any code in this frame."
      }
      frame "API: Test SyncMessage" {
        n94 = call "CSM - Check If Module Exists.vi"("CSM Name"=w228) -> ("error out"=w222:errorcluster, "Exist?"=w223:bool, "CSM Name (Dup)"=w227:string)  [unwired: 8 in]
        n95 = case shown="True" w223 {
          tunnel: w227 -> [_ w231]
          tunnel: [_ w230] -> w224
          frame False {
          }
          frame True {
            n96 = call "uuid.vi"() -> ("UUID"=w232:string)  [unwired: 11 in]
            n97 = call-poly "Build Message with Arguments++.vi"("State With Arguments"="Message", "Arguments (\"\")"=w232, "Target Module (\"\")"=w231) -> ("CSM Message String"=w230:string)  [unwired: 12 in]
          }
        }
        n98 = call <vilib>:"Add State(s) to Queue__JKI_lib_State_Machine.vi"("State(s) in Front (\"\")"=w224, "State(s) in (\"\")"=w225) -> ("States Out"=w226:string)  [unwired: 13 in]
      }
      frame "API: Test SyncMessage With Error" {
        n99 = call "CSM - Check If Module Exists.vi"("CSM Name"=w240) -> ("error out"=w234:errorcluster, "Exist?"=w235:bool, "CSM Name (Dup)"=w239:string)  [unwired: 8 in]
        n100 = case shown="True" w235 {
          tunnel: w239 -> [_ w243]
          tunnel: [_ w242] -> w236
          frame False {
          }
          frame True {
            n101 = call "uuid.vi"() -> ("UUID"=w244:string)  [unwired: 11 in]
            n102 = call "Build Synchronous Message with Arguments.vi"("State With Arguments"="Message With Error", "Arguments (\"\")"=w244, "Target Module (\"\")"=w243) -> ("CSM Message String"=w242:string)  [unwired: 12 in]
          }
        }
        n103 = call <vilib>:"Add State(s) to Queue__JKI_lib_State_Machine.vi"("State(s) in Front (\"\")"=w236, "State(s) in (\"\")"=w237) -> ("States Out"=w238:string)  [unwired: 13 in]
      }
      frame "API: Test SyncMessage via API" {
        n104 = call "CSM - Check If Module Exists.vi"("CSM Name"=w265) -> ("error out"=w260:errorcluster, "Exist?"=w261:bool, "CSM Name (Dup)"=w264:string)  [unwired: 8 in]
        n105 = case shown="True" w261 {
          tunnel: w264 -> [_ w273]
          tunnel: [_ w272] -> w248
          tunnel: w250 -> [_ w271]
          tunnel: [_ w270] -> w257
          tunnel: [_ w269] -> w247
          tunnel: [_ w268] -> w253
          tunnel: [_ w267] -> w256
          frame False {
          }
          frame True {
            w270 = "Message" ("State With Arguments")
            n106 = call "uuid.vi"() -> ("UUID"=w268:string)  [unwired: 11 in]
            n107 = call "CSM - Wait and Send Message for Reply.vi"("State"=w270, "Current Module (\"\" to Generate an ID)"=w271, "Arguments (\"\")"=w268, "Target Module"=w273) -> ("Response"=w267:string, "Source CSM"=w269:string, "error out"=w272:errorcluster)  [unwired: 8 in, 1 out]
          }
        }
        n108 = call "CSM - Resolve Node Module.vi"("Node Name"=w250) -> ("CSM Module Name"=w249:string)  [unwired: 10 in]
        n109 = call "CSM - Resolve Node Module.vi"("Node Name"=w247) -> ("CSM Module Name"=w246:string)  [unwired: 10 in]
        n110 = Bundle By Name(cluster=T1 {"Arguments"="", "Response"="", "error"={"status"=FALSE, "code"=0, "source"=""}}, "Arguments"=w253, "Response"=w256, "error"=w248) -> (w251:T1)
        n111 = Concatenate Strings(w246, ":" ("string"), w257) -> (w255:string)
        n112 = call "CSM - Set Module Attribute.vi"("CSM Name"=w249, "Attribute"=w255, "Value"=w251) -> ("error out"=w254:errorcluster)  [unwired: 9 in, 3 out]
        n113 = call <vilib>:"Add State(s) to Queue__JKI_lib_State_Machine.vi"("State(s) in (\"\")"=w262) -> ("States Out"=w263:string)  [unwired: 14 in]
        n114 = Merge Errors(w254, w248, w260) -> (w259:errorcluster)
      }
      frame "API: Test SyncMessage With Error via API" {
        n115 = call "CSM - Check If Module Exists.vi"("CSM Name"=w293) -> ("error out"=w288:errorcluster, "Exist?"=w289:bool, "CSM Name (Dup)"=w292:string)  [unwired: 8 in]
        n116 = case shown="True" w289 {
          tunnel: w292 -> [_ w301]
          tunnel: [_ w300] -> w276
          tunnel: w278 -> [_ w299]
          tunnel: [_ w298] -> w285
          tunnel: [_ w297] -> w275
          tunnel: [_ w296] -> w281
          tunnel: [_ w295] -> w284
          frame False {
          }
          frame True {
            w298 = "Message With Error" ("State With Arguments")
            n117 = call "uuid.vi"() -> ("UUID"=w296:string)  [unwired: 11 in]
            n118 = call "CSM - Wait and Send Message for Reply.vi"("State"=w298, "Current Module (\"\" to Generate an ID)"=w299, "Arguments (\"\")"=w296, "Target Module"=w301) -> ("Response"=w295:string, "Source CSM"=w297:string, "error out"=w300:errorcluster)  [unwired: 8 in, 1 out]
          }
        }
        n119 = call "CSM - Resolve Node Module.vi"("Node Name"=w275) -> ("CSM Module Name"=w274:string)  [unwired: 10 in]
        n120 = Bundle By Name(cluster=T1 {"Arguments"="", "Response"="", "error"={"status"=FALSE, "code"=0, "source"=""}}, "Arguments"=w281, "Response"=w284, "error"=w276) -> (w280:T1)
        n121 = call "CSM - Resolve Node Module.vi"("Node Name"=w278) -> ("CSM Module Name"=w277:string)  [unwired: 10 in]
        n122 = Concatenate Strings(w274, ":" ("string"), w285) -> (w283:string)
        n123 = call "CSM - Set Module Attribute.vi"("CSM Name"=w277, "Attribute"=w283, "Value"=w280) -> ("error out"=w282:errorcluster)  [unwired: 9 in, 3 out]
        n124 = call <vilib>:"Add State(s) to Queue__JKI_lib_State_Machine.vi"("State(s) in (\"\")"=w290) -> ("States Out"=w291:string)  [unwired: 14 in]
        n125 = Merge Errors(w282, w276, w288) -> (w287:errorcluster)
      }
      frame "API: Test AsyncMessageWithReply" {
        n126 = call "CSM - Check If Module Exists.vi"("CSM Name"=w308) -> ("error out"=w302:errorcluster, "Exist?"=w303:bool, "CSM Name (Dup)"=w307:string)  [unwired: 8 in]
        n127 = case shown="True" w303 {
          tunnel: w307 -> [_ w311]
          tunnel: [_ w310] -> w304
          frame False {
          }
          frame True {
            n128 = call "uuid.vi"() -> ("UUID"=w312:string)  [unwired: 11 in]
            n129 = call-poly "Build Message with Arguments++.vi"("State With Arguments"="Message", "Arguments (\"\")"=w312, "Target Module (\"\")"=w311) -> ("CSM Message String"=w310:string)  [unwired: 12 in]
          }
        }
        n130 = call <vilib>:"Add State(s) to Queue__JKI_lib_State_Machine.vi"("State(s) in Front (\"\")"=w304, "State(s) in (\"\")"=w305) -> ("States Out"=w306:string)  [unwired: 13 in]
      }
      frame "API: Test AsyncMessageWithReply With Error" {
        n131 = call "CSM - Check If Module Exists.vi"("CSM Name"=w320) -> ("error out"=w314:errorcluster, "Exist?"=w315:bool, "CSM Name (Dup)"=w319:string)  [unwired: 8 in]
        n132 = case shown="True" w315 {
          tunnel: w319 -> [_ w324]
          tunnel: [_ w322] -> w316
          frame False {
          }
          frame True {
            n133 = call "uuid.vi"() -> ("UUID"=w323:string)  [unwired: 11 in]
            n134 = call-poly "Build Message with Arguments++.vi"("State With Arguments"="Message With Error", "Arguments (\"\")"=w323, "Target Module (\"\")"=w324) -> ("CSM Message String"=w322:string)  [unwired: 12 in]
          }
        }
        n135 = call <vilib>:"Add State(s) to Queue__JKI_lib_State_Machine.vi"("State(s) in Front (\"\")"=w316, "State(s) in (\"\")"=w317) -> ("States Out"=w318:string)  [unwired: 13 in]
      }
      frame "API: Test AsyncMessageWithoutReply" {
        n136 = call "CSM - Check If Module Exists.vi"("CSM Name"=w332) -> ("error out"=w326:errorcluster, "Exist?"=w327:bool, "CSM Name (Dup)"=w331:string)  [unwired: 8 in]
        n137 = case shown="True" w327 {
          tunnel: w331 -> [_ w337]
          tunnel: [_ w335] -> w328
          frame False {
          }
          frame True {
            n138 = call-poly "Build Message with Arguments++.vi"("State With Arguments"="AsyncMessageWithoutReply", "Arguments (\"\")"="123456789" ("Arguments (\"\")"), "Target Module (\"\")"=w337) -> ("CSM Message String"=w335:string)  [unwired: 12 in]
          }
        }
        n139 = call <vilib>:"Add State(s) to Queue__JKI_lib_State_Machine.vi"("State(s) in Front (\"\")"=w328, "State(s) in (\"\")"=w329) -> ("States Out"=w330:string)  [unwired: 13 in]
      }
      frame "API: Test AsyncMessageWithoutReply via API" {
        n140 = call "CSM - Check If Module Exists.vi"("CSM Name"=w346) -> ("error out"=w341:errorcluster, "Exist?"=w342:bool, "CSM Name (Dup)"=w345:string)  [unwired: 8 in]
        n141 = case shown="True" w342 {
          tunnel: w345 -> [_ w349]
          tunnel: w340 -> [_ w352]
          tunnel: [_ w348] -> w338
          frame False {
          }
          frame True {
            n142 = call "CSM - Wait and Post Message.vi"("State"="AsyncMessageWithoutReply" ("State With Arguments"), "Current Module (\"\" to Generate an ID)"=w352, "Arguments (\"\")"="123456789" ("Arguments (\"\")"), "Target Module"=w349) -> ("error out"=w348:errorcluster)  [unwired: 10 in, 1 out]
          }
        }
        n143 = call <vilib>:"Add State(s) to Queue__JKI_lib_State_Machine.vi"("State(s) in (\"\")"=w343) -> ("States Out"=w344:string)  [unwired: 14 in]
        n144 = Merge Errors(w338, w341) -> (w339:errorcluster)
      }
      frame "API: Test Argument" {
        n145 = call "uuid.vi"() -> ("UUID"=w358:string)  [unwired: 11 in]
        n146 = call "CSM - Convert HexStr to Data.vi"("HEX String"=w362) -> ("Variant"=w360:variant, "error out"=w361:errorcluster)  [unwired: 7 in]
        n147 = Bundle("", "UUID"=w358) -> (w356:cluster{string, "UUID":string})  [unwired: 1 in]
        n148 = Variant To Data(error in=w361, type=w356, Variant=w360) -> (data=w355:cluster{string, "UUID":string}, error out=w359:errorcluster)
        n149 = Unbundle(w355) -> (w354:string, "UUID"=w353:string)
        n150 = call "CSM - Check If Module Exists.vi"("Error In"=w359, "CSM Name"=w354) -> ("error out"=w363:errorcluster, "Exist?"=w364:bool, "CSM Name (Dup)"=w368:string)  [unwired: 7 in]
        n151 = case shown="True" w364 {
          tunnel: w368 -> [_ w372]
          tunnel: [_ w371] -> w365
          tunnel: w353 -> [_ w370]
          frame False {
          }
          frame True {
            n152 = call "Build Synchronous Message with Arguments.vi"("State With Arguments"="ArgumentTest", "Arguments (\"\")"=w370, "Target Module (\"\")"=w372) -> ("CSM Message String"=w371:string)  [unwired: 12 in]
          }
        }
        n153 = call <vilib>:"Add State(s) to Queue__JKI_lib_State_Machine.vi"("State(s) in Front (\"\")"=w365, "State(s) in (\"\")"=w366) -> ("States Out"=w367:string)  [unwired: 13 in]
      }
      frame "API: Test Argument Only For Chain4", "API: Test Argument Only For Chain4And5", "API: Test Argument Only For Chain4And5And6", "API: Test Argument Only For Chain4And6", "API: Test Argument Only For Chain5", "API: Test Argument Only For Chain5And6", "API: Test Argument Only For Chain6" {
        n154 = call "uuid.vi"() -> ("UUID"=w392:string)  [unwired: 11 in]
        n155 = call "CSM - Convert HexStr to Data.vi"("HEX String"=w396) -> ("Variant"=w394:variant, "error out"=w395:errorcluster)  [unwired: 7 in]
        n156 = Match Pattern(string=w380, regular expression="Chain") -> (after substring=w375:string, offset past match=w378:i32)  [unwired: 1 in, 2 out]
        n157 = Bundle("", "UUID"=w392) -> (w390:cluster{string, "UUID":string})  [unwired: 1 in]
        n158 = Variant To Data(error in=w395, type=w390, Variant=w394) -> (data=w389:cluster{string, "UUID":string}, error out=w393:errorcluster)
        n159 = Not Equal?(x=w378, y=-1) -> (x != y?=w376:bool)
        n160 = call "CSM - Resolve Node Module.vi"("Node Name"=w386) -> ("CSM Module Name"=w385:string)  [unwired: 10 in]
        n161 = case shown="True" w376 {
          tunnel: w375 -> [_ w402]
          tunnel: [_ w402] -> w374
          frame False {
          }
          frame True {
          }
        }
        n162 = Unbundle(w389) -> (w388:string, "UUID"=w387:string)
        n163 = call "CSM - Check If Module Exists.vi"("Error In"=w393, "CSM Name"=w388) -> ("error out"=w384:errorcluster, "Exist?"=w397:bool, "CSM Name (Dup)"=w400:string)  [unwired: 7 in]
        n164 = case shown="True" w397 {
          tunnel: w400 -> [_ w409]
          tunnel: w387 -> [_ w410]
          tunnel: [_ w408] -> w381
          tunnel: w385 -> [_ w407]
          tunnel: [_ w406] -> w383
          tunnel: w374 -> [_ w404]
          frame False {
          }
          frame True {
            n165 = Concatenate Strings("ArgumentTestOnlyForChain" ("State With Arguments"), w404) -> (w403:string)
            n166 = call "CSM - Wait and Send Message for Reply.vi"("State"=w403, "Current Module (\"\" to Generate an ID)"=w407, "Arguments (\"\")"=w410, "Target Module"=w409) -> ("Response"=w406:string, "error out"=w408:errorcluster)  [unwired: 8 in, 2 out]
          }
        }
        n167 = call <vilib>:"Add State(s) to Queue__JKI_lib_State_Machine.vi"("State(s) in (\"\")"=w398) -> ("States Out"=w399:string)  [unwired: 14 in]
        n168 = Merge Errors(w384, w381) -> (w382:errorcluster)
      }
      frame "API: Test Response With Error" {
        n169 = call "CSM - Check If Module Exists.vi"("CSM Name"=w417) -> ("error out"=w411:errorcluster, "Exist?"=w412:bool, "CSM Name (Dup)"=w416:string)  [unwired: 8 in]
        n170 = case shown="True" w412 {
          tunnel: w416 -> [_ w420]
          tunnel: [_ w419] -> w413
          frame False {
          }
          frame True {
            n171 = call "uuid.vi"() -> ("UUID"=w421:string)  [unwired: 11 in]
            n172 = call "Build Synchronous Message with Arguments.vi"("State With Arguments"="Response With Error", "Arguments (\"\")"=w421, "Target Module (\"\")"=w420) -> ("CSM Message String"=w419:string)  [unwired: 12 in]
          }
        }
        n173 = call <vilib>:"Add State(s) to Queue__JKI_lib_State_Machine.vi"("State(s) in Front (\"\")"=w413, "State(s) in (\"\")"=w414) -> ("States Out"=w415:string)  [unwired: 13 in]
      }
      frame "API: Test MacroWithSubMessages" {
        n174 = call <vilib>:"Build State String with Arguments__JKI_lib_State_Machine.vi"("Arguments (\"\")"=w424, "State"="Macro: Test MacroWithSubMessages") -> ("State with Arguments"=w423:string)  [unwired: 4 in]
        n175 = call <vilib>:"Add State(s) to Queue__JKI_lib_State_Machine.vi"("State(s) in Front (\"\")"=w423, "State(s) in (\"\")"=w427) -> ("States Out"=w426:string)  [unwired: 13 in]
      }
      frame "API: Test MacroWithSubAndPostMessages" {
        n176 = call <vilib>:"Build State String with Arguments__JKI_lib_State_Machine.vi"("Arguments (\"\")"=w431, "State"="Macro: Test MacroWithSubAndPostMessages") -> ("State with Arguments"=w430:string)  [unwired: 4 in]
        n177 = call <vilib>:"Add State(s) to Queue__JKI_lib_State_Machine.vi"("State(s) in Front (\"\")"=w430, "State(s) in (\"\")"=w434) -> ("States Out"=w433:string)  [unwired: 13 in]
      }
      frame "API: Test MacroWithNonLocalSubMessages" {
        n178 = call <vilib>:"Build State String with Arguments__JKI_lib_State_Machine.vi"("Arguments (\"\")"=w438, "State"="Macro: TestMacroWithNonLocalSubMessages") -> ("State with Arguments"=w437:string)  [unwired: 4 in]
        n179 = call <vilib>:"Add State(s) to Queue__JKI_lib_State_Machine.vi"("State(s) in Front (\"\")"=w437, "State(s) in (\"\")"=w441) -> ("States Out"=w440:string)  [unwired: 13 in]
      }
      frame "API: Test Register State" {
        n180 = call <vilib>:"Build State String with Arguments__JKI_lib_State_Machine.vi"("Arguments (\"\")"=w445, "State"="Test Status") -> ("State with Arguments"=w444:string)  [unwired: 4 in]
        n181 = call <vilib>:"Add State(s) to Queue__JKI_lib_State_Machine.vi"("State(s) in Front (\"\")"=w444, "State(s) in (\"\")"=w448) -> ("States Out"=w447:string)  [unwired: 13 in]
      }
      frame "API: Test Register State Argument Info" {
        n182 = call <vilib>:"Build State String with Arguments__JKI_lib_State_Machine.vi"("Arguments (\"\")"=w452, "State"="Register State Argument Info") -> ("State with Arguments"=w451:string)  [unwired: 4 in]
        n183 = call <vilib>:"Add State(s) to Queue__JKI_lib_State_Machine.vi"("State(s) in Front (\"\")"=w451, "State(s) in (\"\")"=w455) -> ("States Out"=w454:string)  [unwired: 13 in]
      }
      frame "API: Test Register Status" {
        n184 = call <vilib>:"Build State String with Arguments__JKI_lib_State_Machine.vi"("Arguments (\"\")"=w459, "State"="Register Status") -> ("State with Arguments"=w458:string)  [unwired: 4 in]
        n185 = call <vilib>:"Add State(s) to Queue__JKI_lib_State_Machine.vi"("State(s) in Front (\"\")"=w458, "State(s) in (\"\")"=w462) -> ("States Out"=w461:string)  [unwired: 13 in]
      }
      frame "API: Test Register Interrupt" {
        n186 = call <vilib>:"Build State String with Arguments__JKI_lib_State_Machine.vi"("Arguments (\"\")"=w466, "State"="Register Interrupt") -> ("State with Arguments"=w465:string)  [unwired: 4 in]
        n187 = call <vilib>:"Add State(s) to Queue__JKI_lib_State_Machine.vi"("State(s) in Front (\"\")"=w465, "State(s) in (\"\")"=w469) -> ("States Out"=w468:string)  [unwired: 13 in]
      }
      frame "API: Test Register Status Argument Info" {
        n188 = call <vilib>:"Build State String with Arguments__JKI_lib_State_Machine.vi"("Arguments (\"\")"=w473, "State"="Register Status Argument Info") -> ("State with Arguments"=w472:string)  [unwired: 4 in]
        n189 = call <vilib>:"Add State(s) to Queue__JKI_lib_State_Machine.vi"("State(s) in Front (\"\")"=w472, "State(s) in (\"\")"=w476) -> ("States Out"=w475:string)  [unwired: 13 in]
      }
      frame "API: Test Status A" {
        n190 = call <vilib>:"Build State String with Arguments__JKI_lib_State_Machine.vi"("Arguments (\"\")"=w480, "State"="Broadcast Status A") -> ("State with Arguments"=w481:string)  [unwired: 4 in]
        n191 = call <vilib>:"Add State(s) to Queue__JKI_lib_State_Machine.vi"("State(s) in Front (\"\")"=w481, "State(s) in (\"\")"=w483) -> ("States Out"=w482:string)  [unwired: 13 in]
      }
      frame "API: Test State A" {
        n192 = call <vilib>:"Build State String with Arguments__JKI_lib_State_Machine.vi"("Arguments (\"\")"=w487, "State"="State A") -> ("State with Arguments"=w488:string)  [unwired: 4 in]
        n193 = call <vilib>:"Add State(s) to Queue__JKI_lib_State_Machine.vi"("State(s) in Front (\"\")"=w488, "State(s) in (\"\")"=w490) -> ("States Out"=w489:string)  [unwired: 13 in]
      }
      frame "API: Test State B" {
        n194 = call <vilib>:"Build State String with Arguments__JKI_lib_State_Machine.vi"("Arguments (\"\")"=w494, "State"="State B") -> ("State with Arguments"=w495:string)  [unwired: 4 in]
        n195 = call <vilib>:"Add State(s) to Queue__JKI_lib_State_Machine.vi"("State(s) in Front (\"\")"=w495, "State(s) in (\"\")"=w497) -> ("States Out"=w496:string)  [unwired: 13 in]
      }
      frame "API: Test Status B" {
        n196 = call <vilib>:"Build State String with Arguments__JKI_lib_State_Machine.vi"("Arguments (\"\")"=w501, "State"="Broadcast Status B") -> ("State with Arguments"=w502:string)  [unwired: 4 in]
        n197 = call <vilib>:"Add State(s) to Queue__JKI_lib_State_Machine.vi"("State(s) in Front (\"\")"=w502, "State(s) in (\"\")"=w504) -> ("States Out"=w503:string)  [unwired: 13 in]
      }
      frame "API: Local Registration" {
        # "Test Status @ From >> Handler Message @ To -><register>"
        n198 = call "CSM - Resolve Node Module.vi"("Node Name"=w511) -> ("CSM Module Name"=w507:string)  [unwired: 10 in]
        n199 = call-poly "Build Message with Arguments++.vi"("Target CSM"=w508, "Source CSM (* as Default)"=w507, "Status"="Test Status", "API (If \"\", Same As \"Status\")"="Handler Message") -> ("CSM Message String"=w509:string)  [unwired: 11 in]
        n200 = call <vilib>:"Add State(s) to Queue__JKI_lib_State_Machine.vi"("State(s) in Front (\"\")"=w509, "State(s) in (\"\")"=w515) -> ("States Out"=w514:string)  [unwired: 13 in]
      }
      frame "API: Local Registration II" {
        # "Test Status @ From >> Handler Message -><register>"
        n201 = call "CSM - Resolve Node Module.vi"("Node Name"=w519) -> ("CSM Module Name"=w516:string)  [unwired: 10 in]
        n202 = call-poly "Build Message with Arguments++.vi"("Source CSM (* as Default)"=w516, "Status"="Test Status", "API (If \"\", Same As \"Status\")"="Handler Message") -> ("CSM Message String"=w517:string)  [unwired: 12 in]
        n203 = call <vilib>:"Add State(s) to Queue__JKI_lib_State_Machine.vi"("State(s) in Front (\"\")"=w517, "State(s) in (\"\")"=w523) -> ("States Out"=w522:string)  [unwired: 13 in]
      }
      frame "API: Local Unregistration" {
        # "Test Status @ From >> Handler Message @ To -><unregister>"
        n204 = call "CSM - Resolve Node Module.vi"("Node Name"=w528) -> ("CSM Module Name"=w524:string)  [unwired: 10 in]
        n205 = call-poly "Build Message with Arguments++.vi"("Target CSM"=w525, "Source CSM (* as Default)"=w524, "Status"="Test Status", "API (If \"\", Same As \"Status\")"="Handler Message") -> ("CSM Message String"=w526:string)  [unwired: 11 in]
        n206 = call <vilib>:"Add State(s) to Queue__JKI_lib_State_Machine.vi"("State(s) in Front (\"\")"=w526, "State(s) in (\"\")"=w532) -> ("States Out"=w531:string)  [unwired: 13 in]
      }
      frame "API: Local Registration via API" {
        # "Test Status @ From >> Handler Message @ To -><register>"
        n207 = call "CSM - Resolve Node Module.vi"("Node Name"=w538) -> ("CSM Module Name"=w534:string)  [unwired: 10 in]
        n208 = call "CSM - Register Broadcast.vi"("CSM Name(Empty for Broadcast Event)"=w533, "Source CSM Name (* as Default)"=w534, "Trigger"="Test Status", "API (If \"\", Same as Trigger)"="Handler Message") -> ("error out"=w537:errorcluster)  [unwired: 10 in, 1 out]
        n209 = call <vilib>:"Add State(s) to Queue__JKI_lib_State_Machine.vi"("State(s) in (\"\")"=w541) -> ("States Out"=w540:string)  [unwired: 14 in]
      }
      frame "API: Local Unregistration via API" {
        # "Test Status @ From >> Handler Message @ To -><unregister>"
        n210 = call "CSM - Resolve Node Module.vi"("Node Name"=w547) -> ("CSM Module Name"=w543:string)  [unwired: 10 in]
        n211 = call "CSM - Unregister Broadcast.vi"("CSM Name(Empty for Broadcast Event)"=w542, "Source CSM Name (* as Default)"=w543, "Trigger"="Test Status", "API (\"*\" as Default)"="Handler Message") -> ("error out"=w546:errorcluster)  [unwired: 10 in, 1 out]
        n212 = call <vilib>:"Add State(s) to Queue__JKI_lib_State_Machine.vi"("State(s) in (\"\")"=w550) -> ("States Out"=w549:string)  [unwired: 14 in]
      }
      frame "API: API2" {
        # "#CSM API Example\nCopy/Rename this case for your own API"
        # "unpack Hex String  to Variant\nif complex parameter is needed."
        n213 = call "CSM - Convert HexStr to Data.vi"("HEX String"=w552) -> ()  [unwired: 7 in, 2 out]
        n214 = disable-structure shown="Enabled" {
          disable-tunnel: [w555 "API2 Response"] -> w551
          frame Disabled {
            # "pack variant to hexstr \nif complex response is needed."
            # "complex Response"
            n215 = call "CSM - Convert Data to HexStr.vi"() -> ("HEX String (0-9,A-F)"=w555:string)  [unwired: 9 in]
          }
          frame Enabled {
          }
        }
      }
      frame "---------- Action ----------" {
        # "#CSM \"Category Seperator\"\nDo not put any code in this frame."
        n216 = call <vilib>:"Add State(s) to Queue__JKI_lib_State_Machine.vi"("State(s) in (\"\")"=w559) -> ("States Out"=w558:string)  [unwired: 14 in]
      }
      frame "Action: action1" {
        # "#CSM \"Internal State\"\nThis category is used for holding internal states"
        n217 = call <vilib>:"Add State(s) to Queue__JKI_lib_State_Machine.vi"("State(s) in (\"\")"=w562) -> ("States Out"=w561:string)  [unwired: 14 in]
      }
      frame "Test Status" {
        n218 = call <vilib>:"Add State(s) to Queue__JKI_lib_State_Machine.vi"("State(s) in (\"\")"=w566) -> ("States Out"=w565:string)  [unwired: 14 in]
      }
      frame "Register State Argument Info" {
        n219 = call "CSM - Resolve Node Module.vi"("Node Name"=w569) -> ("CSM Module Name"=w570:string)  [unwired: 10 in]
        n220 = Concatenate Strings(w567, "+", w570) -> (w568:string)
        n221 = call <vilib>:"Add State(s) to Queue__JKI_lib_State_Machine.vi"("State(s) in (\"\")"=w572) -> ("States Out"=w574:string)  [unwired: 14 in]
      }
      frame "Register Status" {
        n222 = call <vilib>:"Build State String with Arguments__JKI_lib_State_Machine.vi"("Arguments (\"\")"=w575, "State"="Test Status") -> ("State with Arguments"=w577:string)  [unwired: 4 in]
        n223 = call "CSM - Broadcast Status Change.vi"("Status With Arguments"=w577, "State Queue"=w579) -> ("Remaining States"=w576:string)  [unwired: 13 in]
      }
      frame "Register Interrupt" {
        n224 = call-poly "Build Message with Arguments++.vi"("State With Arguments"="Test Interrupt", "Arguments (\"\")"=w584) -> ("CSM Message String"=w583:string)  [unwired: 13 in]
        n225 = call <vilib>:"Add State(s) to Queue__JKI_lib_State_Machine.vi"("State(s) in Front (\"\")"=w583, "State(s) in (\"\")"=w582) -> ("States Out"=w581:string)  [unwired: 13 in]
      }
      frame "Register Status Argument Info" {
        w591 = "Test Status Argument Info"
        n226 = call "CSM - Resolve Node Module.vi"("Node Name"=w589) -> ("CSM Module Name"=w588:string)  [unwired: 10 in]
        n227 = Concatenate Strings(w591, "+", w588) -> (w587:string)
        n228 = call <vilib>:"Build State String with Arguments__JKI_lib_State_Machine.vi"("Arguments (\"\")"=w587, "State"=w591) -> ("State with Arguments"=w593:string)  [unwired: 4 in]
        n229 = call "CSM - Broadcast Status Change.vi"("Status With Arguments"=w593, "State Queue"=w594) -> ("Remaining States"=w592:string)  [unwired: 13 in]
      }
      frame "Broadcast Status A" {
        n230 = call <vilib>:"Build State String with Arguments__JKI_lib_State_Machine.vi"("Arguments (\"\")"=w596, "State"="Status A") -> ("State with Arguments"=w598:string)  [unwired: 4 in]
        n231 = call "CSM - Broadcast Status Change.vi"("Status With Arguments"=w598, "State Queue"=w600) -> ("Remaining States"=w597:string)  [unwired: 13 in]
      }
      frame "Broadcast Status B" {
        n232 = call <vilib>:"Build State String with Arguments__JKI_lib_State_Machine.vi"("Arguments (\"\")"=w602, "State"="Status B") -> ("State with Arguments"=w604:string)  [unwired: 4 in]
        n233 = call "CSM - Broadcast Status Change.vi"("Status With Arguments"=w604, "State Queue"=w606) -> ("Remaining States"=w603:string)  [unwired: 13 in]
      }
      frame "State A" {
        n234 = call <vilib>:"Add State(s) to Queue__JKI_lib_State_Machine.vi"("State(s) in (\"\")"=w610) -> ("States Out"=w609:string)  [unwired: 14 in]
      }
      frame "State B" {
        n235 = call <vilib>:"Add State(s) to Queue__JKI_lib_State_Machine.vi"("State(s) in (\"\")"=w615) -> ("States Out"=w614:string)  [unwired: 14 in]
      }
      frame "Message" {
      }
      frame "SubMessage1" {
      }
      frame "SubMessage2" {
      }
      frame "SubMessage3" {
        n236 = call "CSM - Resolve Node Module.vi"("Node Name"=w635) -> ("CSM Module Name"=w634:string)  [unwired: 10 in]
        n237 = call "CSM - Set Module Attribute.vi"("CSM Name"=w634, "Attribute"=w633, "Value"=w632) -> ("error out"=w630:errorcluster)  [unwired: 9 in, 3 out]
        n238 = Merge Errors(w630, w638) -> (w631:errorcluster)
      }
      frame "PostMessage1" {
      }
      frame "Message With Error" {
        n239 = Merge Errors(errorcluster {"status"=TRUE, "code"=1234567898, "source"="Simulated Error\nwill be sent to Response case"} ("error out"), w644) -> (w643:errorcluster)
      }
      frame "Response With Error" {
        n240 = Merge Errors(errorcluster {"status"=TRUE, "code"=1234567898, "source"="Simulated Error"} ("error out"), w650) -> (w649:errorcluster)
      }
      frame "ArgumentTest" {
        n241 = call "CSM - Resolve Node Module.vi"("Node Name"=w660) -> ("CSM Module Name"=w659:string)  [unwired: 10 in]
        n242 = call "CSM - Set Module Attribute.vi"("CSM Name"=w659, "Attribute"=w657, "Value"=w658) -> ("error out"=w655:errorcluster)  [unwired: 9 in, 3 out]
        n243 = Merge Errors(w655, w663) -> (w656:errorcluster)
      }
      frame "ArgumentTestOnlyForChain4", "ArgumentTestOnlyForChain4And5", "ArgumentTestOnlyForChain4And5And6", "ArgumentTestOnlyForChain4And6", "ArgumentTestOnlyForChain5", "ArgumentTestOnlyForChain5And6", "ArgumentTestOnlyForChain6" {
        n244 = call "CSM - Resolve Node Module.vi"("Node Name"=w664) -> ("CSM Module Name"=w669:string)  [unwired: 10 in]
        n245 = call "CSM - Set Module Attribute.vi"("CSM Name"=w669, "Attribute"=w664, "Value"=w664) -> ("error out"=w666:errorcluster)  [unwired: 9 in, 3 out]
        n246 = Merge Errors(w666, w671) -> (w668:errorcluster)
      }
      frame "AsyncMessageWithoutReply" {
        # "123456789 string constant"
        n247 = call "CSM - Resolve Node Module.vi"("Node Name"=w675) -> ("CSM Module Name"=w674:string)  [unwired: 10 in]
        n248 = call "CSM - Set Module Attribute.vi"("CSM Name"=w674, "Attribute"=w676, "Value"=w677) -> ("error out"=w672:errorcluster)  [unwired: 9 in, 3 out]
        n249 = Merge Errors(w672, w680) -> (w673:errorcluster)
      }
      frame "Handler Message" {
        n250 = call "CSM - Resolve Node Module.vi"("Node Name"=w686) -> ("CSM Module Name"=w685:string)  [unwired: 10 in]
        n251 = call "CSM - Set Module Attribute.vi"("CSM Name"=w685, "Attribute"=w683, "Value"=w682) -> ("error out"=w681:errorcluster)  [unwired: 9 in, 3 out]
        n252 = Merge Errors(w689, w681) -> (w684:errorcluster)
      }
      frame "Handler Message With Counter" {
        n253 = Unbundle By Name(w695) -> ("Counter"=w696:u32)
        n254 = Decimal String To Number(string=w693) -> (number=w690:i32)  [unwired: 2 in, 1 out]
        n255 = Increment(x=w696) -> (x+1=w691:u32)
        n256 = Bundle By Name(cluster=w695, "Counter"=w691) -> (w694:T6)
        n257 = Equal?(x=w691, y=w690) -> (x = y?=w692:bool)
        n258 = call "CSM - Resolve Node Module.vi"("Node Name"=w701) -> ("CSM Module Name"=w700:string)  [unwired: 10 in]
        n259 = case shown="False" w692 {
          tunnel: w700 -> [_ w707]
          tunnel: w698 -> [_ w706]
          tunnel: [_ w705] -> w697
          tunnel: w691 -> [_ w704]
          frame False {
          }
          frame True {
            n260 = call "CSM - Set Module Attribute.vi"("CSM Name"=w707, "Attribute"=w706, "Value"=w704) -> ("error out"=w705:errorcluster)  [unwired: 9 in, 3 out]
          }
        }
        n261 = Merge Errors(w703, w697) -> (w699:errorcluster)
      }
      frame "Reset Counter" {
        # "#CSM \"Internal State\"\nThis category is used for holding internal states"
        n262 = Bundle By Name(cluster=w710, "Counter"=u32 0) -> (w708:T6)
        n263 = call <vilib>:"Add State(s) to Queue__JKI_lib_State_Machine.vi"("State(s) in (\"\")"=w712) -> ("States Out"=w711:string)  [unwired: 14 in]
      }
    }
  }
